vi "DimostratoreTest.vi"() -> ()   [LabVIEW 2019]
doc: "Dimostratore API\n\nFunzionamento:\n1. Seleziona postazione e data\n Conferma\n Ottieni un array con tutti i test della postazione selezionata in base alla data\n2. Seleziona quale test eseguire\n Conferma che tutti gli assets dei test sono disponibili\n Mostra tutti gli step di un test\n3. Seleziona Step da eseguire inserendo anche un valore di prova\n Il risultato dello step viene riprodotto nell'outcome\n\nFunzionamento alternativo\n1. Imposta uno Step Id e conferma\n2. Inserisci un valore di prova e ottieni l'outcome"
uses:
  ByteGSAPIBase/ByteGSAPIBase.lvclass
  TypeDef/MachineStates.ctl
  ByteGSAPIBase/TypeDef/Test.ctl
  ByteGSAPIBase/TypeDef/Asset.ctl
  ByteGSAPIBase/TypeDef/Step.ctl
  <vilib>/Utility/miscctls.llb/LVStringsAndValuesArrayTypeDef_I32.ctl
panel:
  in  "Exit":bool=TRUE
  out "Step Name":string
  in  "Home":bool
  in  "Indietro":bool
  out "Infos":string
  in  "Duration":dbl
  in  "Ottieni Passaggio Step":bool
  in  "Step Id":i32
  in  "Valore Prova":dbl
  in  "Inizia Step":bool
  in  "Seleziona Step":i32(ring) items=["Prova di durata"=23]
  in  "Inizia Test":bool
  in  "Seleziona Test":i32(ring)
  out "error out":errorcluster
  in  "error in (no error)":errorcluster
  in  "Ottieni Test Per Postazione":bool
  in  "ByteGSAPIBase in":refnum<class "ByteGSAPIBase.lvclass">
  in  "Data Partenza":timestamp format="%<%x>T"
  in  "Postazione":enum16{"POST 1", "POST 2"}(ring)
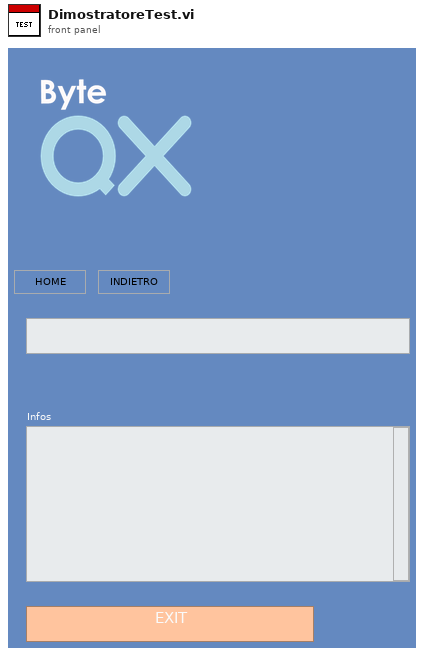
[diagram p1: front panel]
types:
  T1 = typedef "ByteGSWebAPI.lvlib/ByteGSAPIBase.lvclass/Step.ctl" = cluster{"id":i32, "descrizione":string, "prova":string, "assets":T2[], "criterio_accettazione":string, "valore_criterio_accettazione_max":dbl, "valore_criterio_accettazione_min":dbl, "udm_criterio_accettazione":string, "duration_prova":string, "udm_duration_prova":string, "valore_prova":dbl, "ordine":i32, "user":i32, "link_automation":string, "instruction_automation":string, "data_completamento_checklist":timestamp, "outcome":bool}
  T2 = typedef "ByteGSWebAPI.lvlib/ByteGSAPIBase.lvclass/Asset.ctl" = cluster{"descrizione":string, "slug":string, "id":i32}
  T3 = typedef "ByteGSWebAPI.lvlib/ByteGSAPIBase.lvclass/Test.ctl" = cluster{"titolo":string, "descrizione":string, "statoprova":string, "assets":T2[], "id":i32, "data_apertura_prova":timestamp}
  T4 = typedef "MachineStates.ctl" = enum16{"Initialize", "Idle", "GetLimsTestsForBench", "AssetsCheck", "GetLimsTestSteps", "UpdateLimsTestStep", "GetLimsTestStep", "Indietro", "UpdateLimsTestStepAutomation"}
  T5 = cluster{"Postazione":refnum<vi>, "Data Partenza":refnum<vi>, "Ottieni Test Per Postazione":refnum<vi>, "Step Id":refnum<vi>, "Ottieni Passaggio Step":refnum<vi>, "Seleziona Test":refnum<vi>, "Inizia Test":refnum<vi>, "Seleziona Step":refnum<vi>, "Valore Prova":refnum<vi>, "Inizia Step":refnum<vi>, "Infos":refnum<vi>, "Duration":refnum<vi>, "Step Name":refnum<vi>, "Exit":refnum<vi>}
  T6 = cluster{"ByteGSAPIBase in":refnum<class "ByteGSAPIBase.lvclass">, "Array dei Test":T3[], "Steps Array":T1[]}
  T7 = typedef "LVStringsAndValuesArrayTypeDef_I32.ctl" = cluster{"String":string, "Value":i32}[]
  T8 = cluster{"Postazione":enum16{"POST 1", "POST 2"}, "Data Partenza":timestamp, "Seleziona Test":i32, "Seleziona Step":i32, "Valore Prova":dbl, "Step Id":i32, "Duration":dbl}
  T9 = typedef "ByteGSWebAPI.lvlib/ByteGSAPIBase.lvclass/UpdateLimsTestStepData.ctl" = cluster{"outcome":bool, "data_completamento_checklist":timestamp, "udm_duration_prova":string, "valore_prova":dbl, "link_automation":string, "instruction_automation":string, "duration_prova":string}
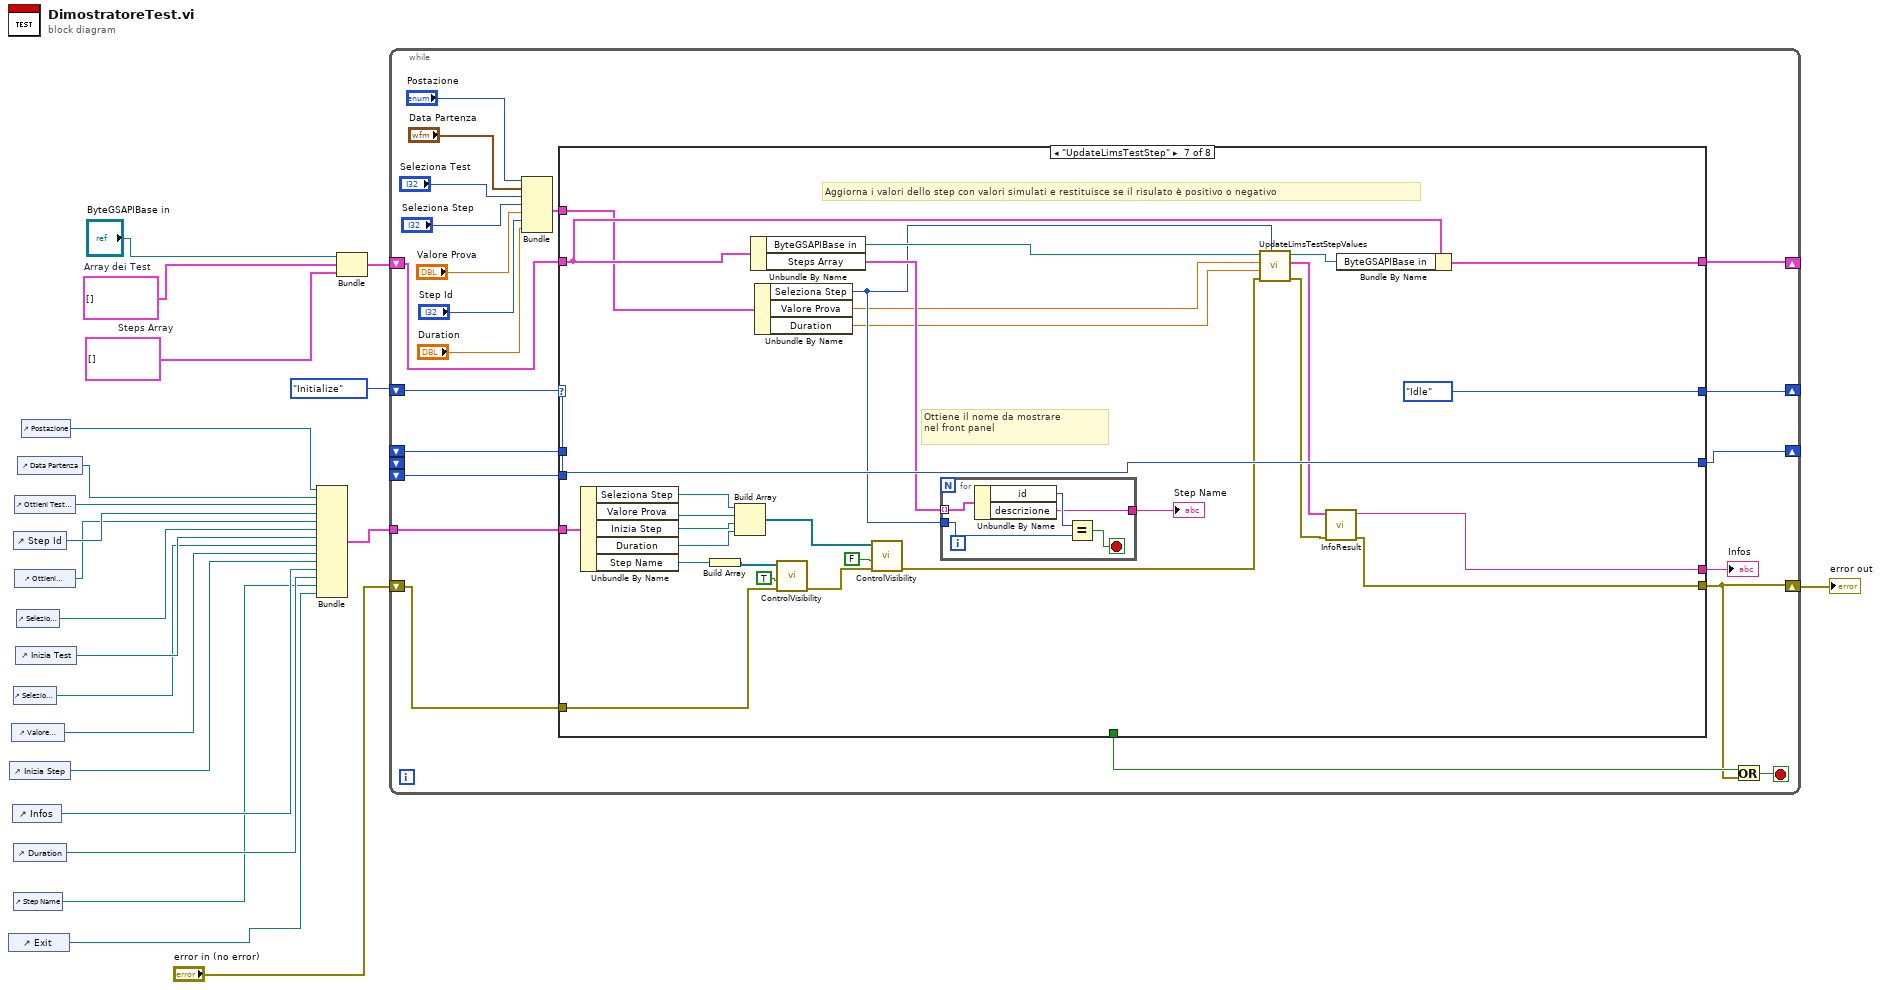
[diagram p0: block diagram]
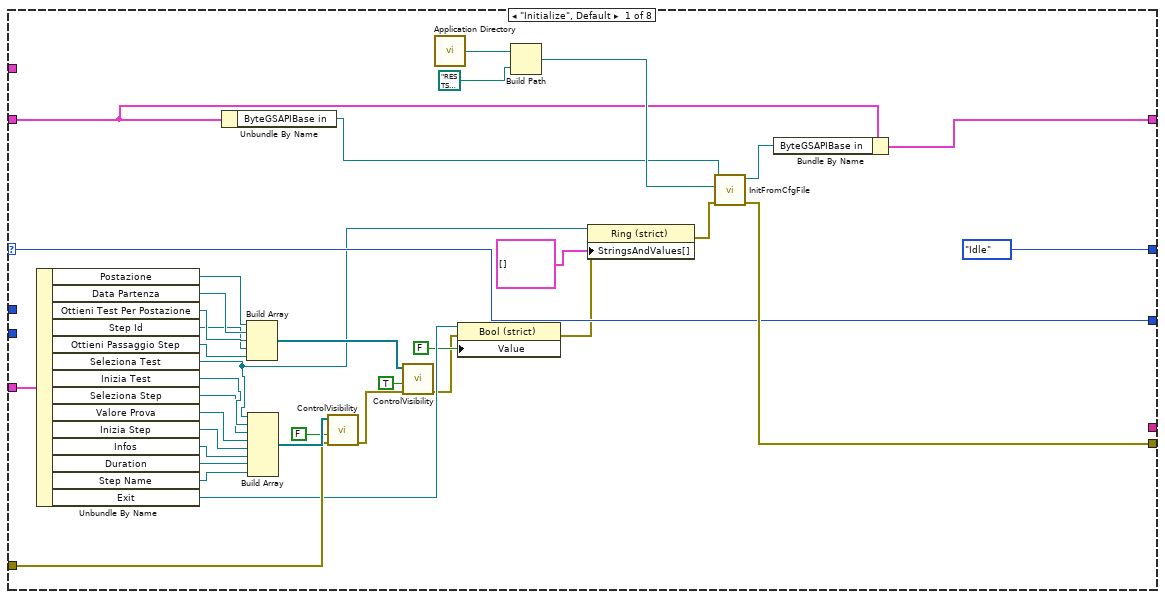
[diagram p2: hidden frame]
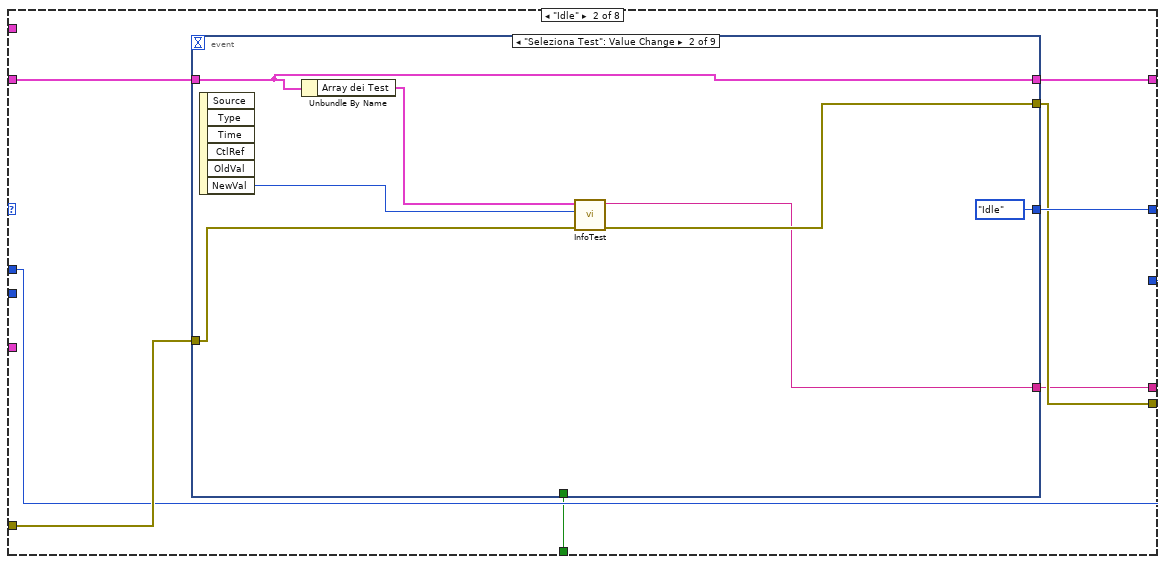
[diagram p3: hidden frame]
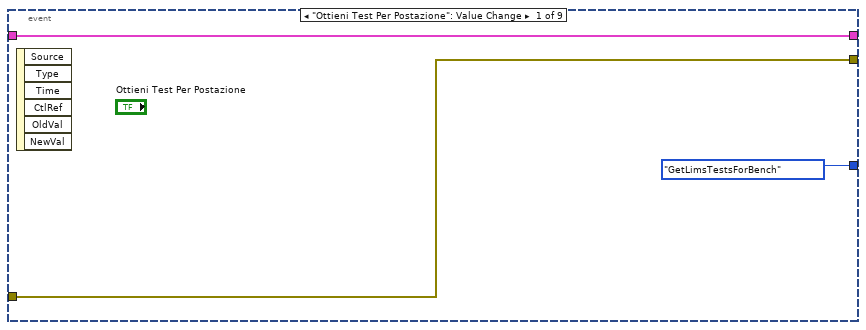
[diagram p4: hidden frame]
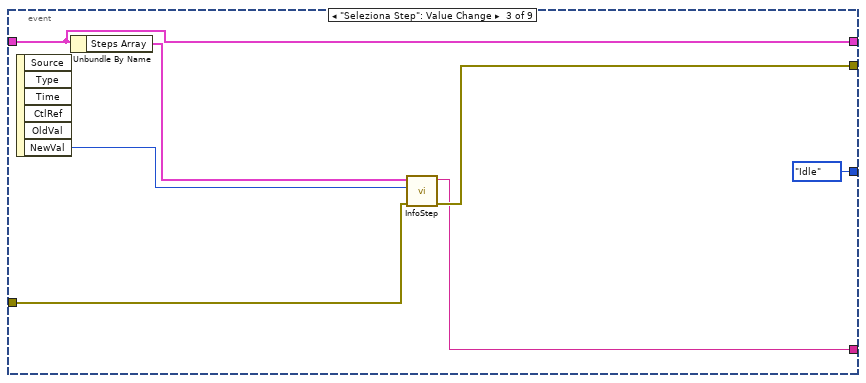
[diagram p5: hidden frame]
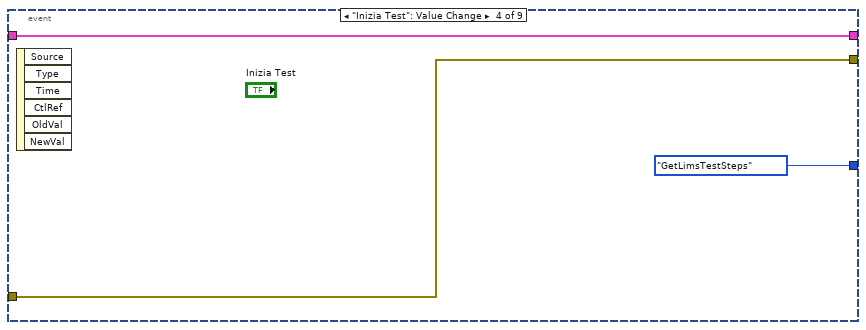
[diagram p6: hidden frame]
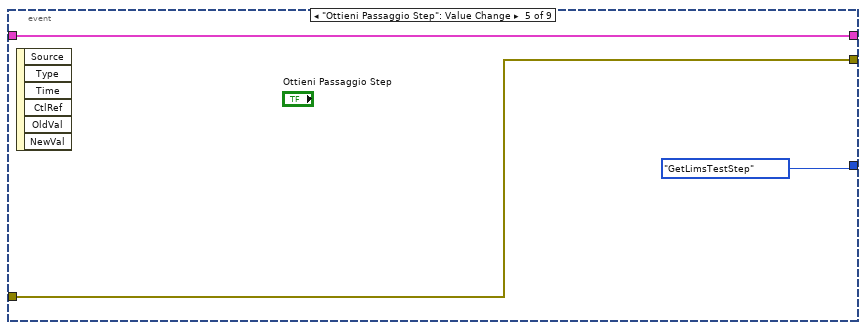
[diagram p7: hidden frame]
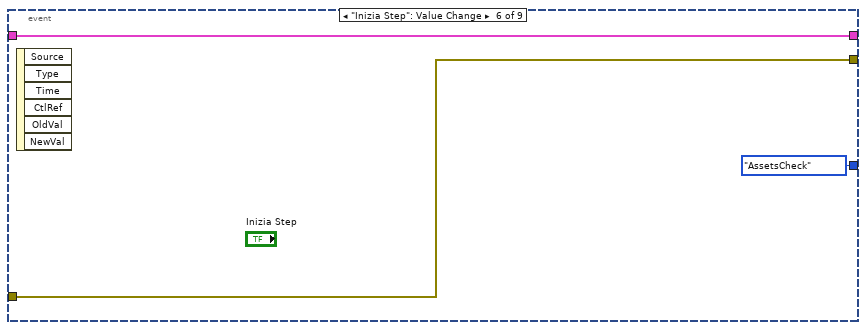
[diagram p8: hidden frame]
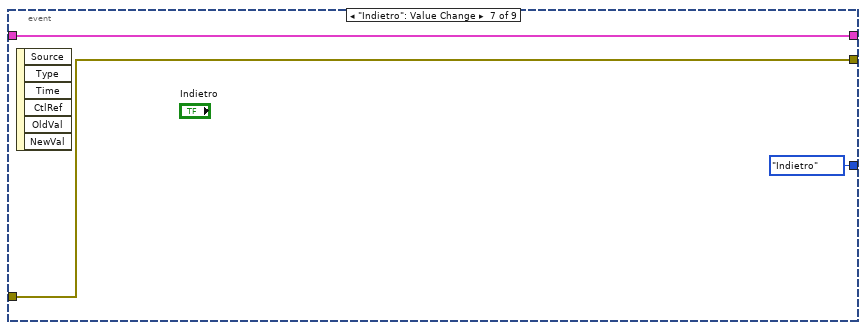
[diagram p9: hidden frame]
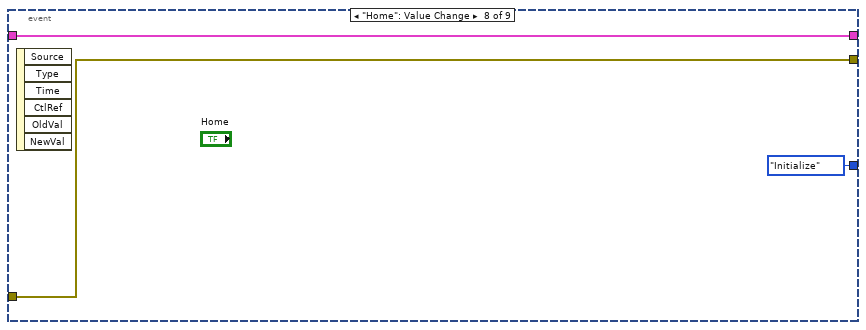
[diagram p10: hidden frame]
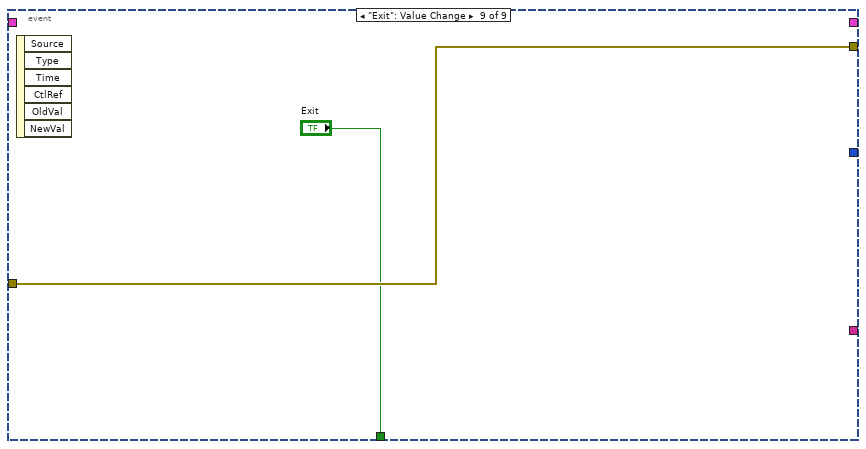
[diagram p11: hidden frame]
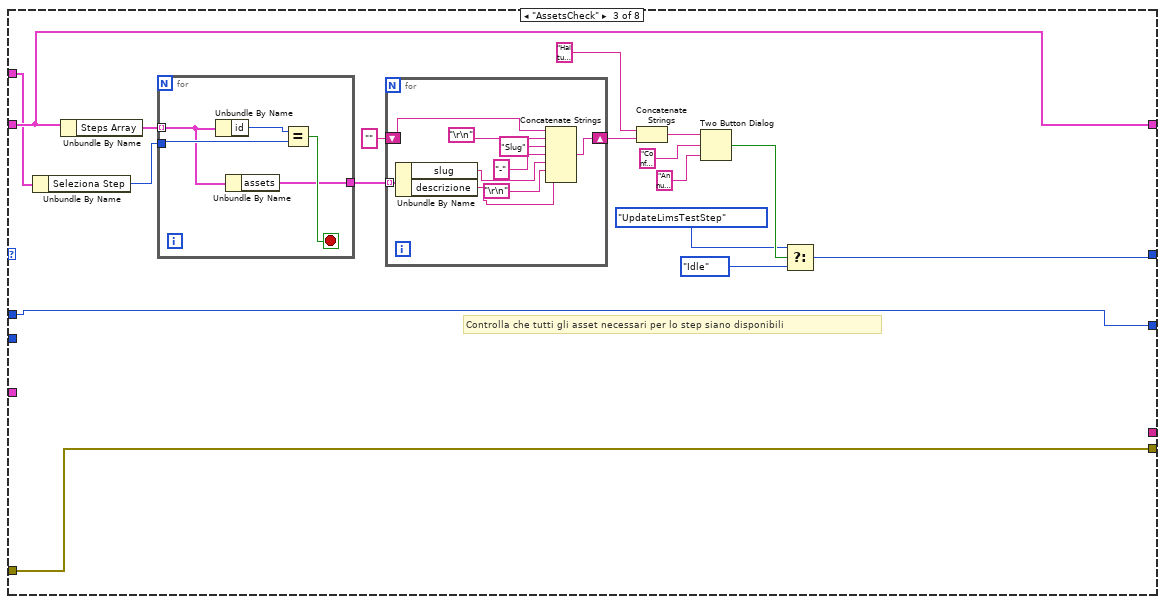
[diagram p12: hidden frame]
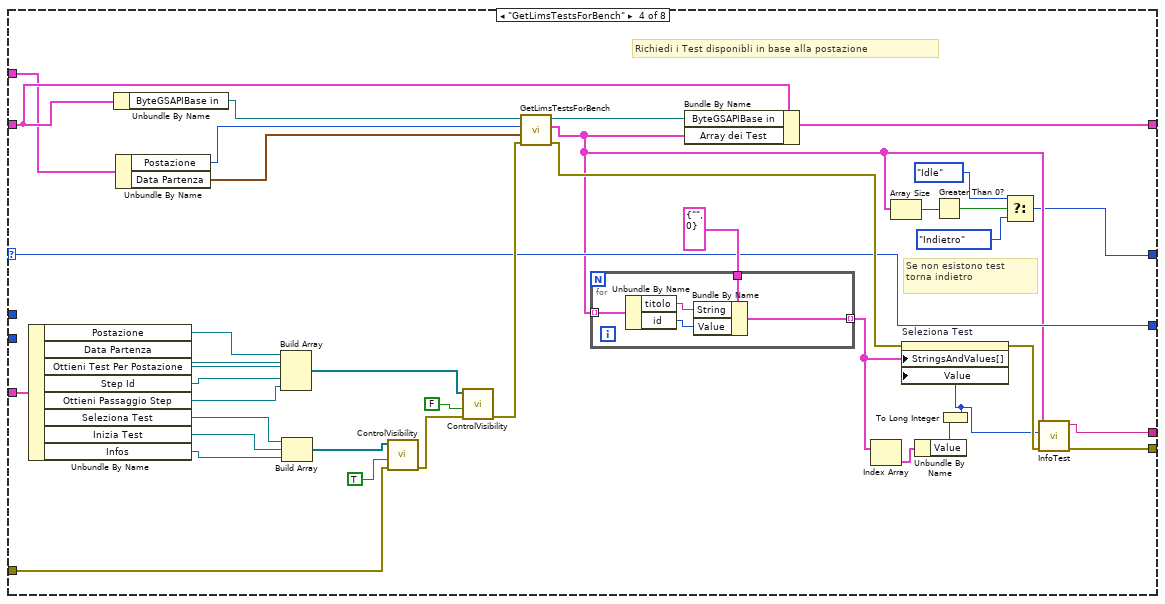
[diagram p13: hidden frame]
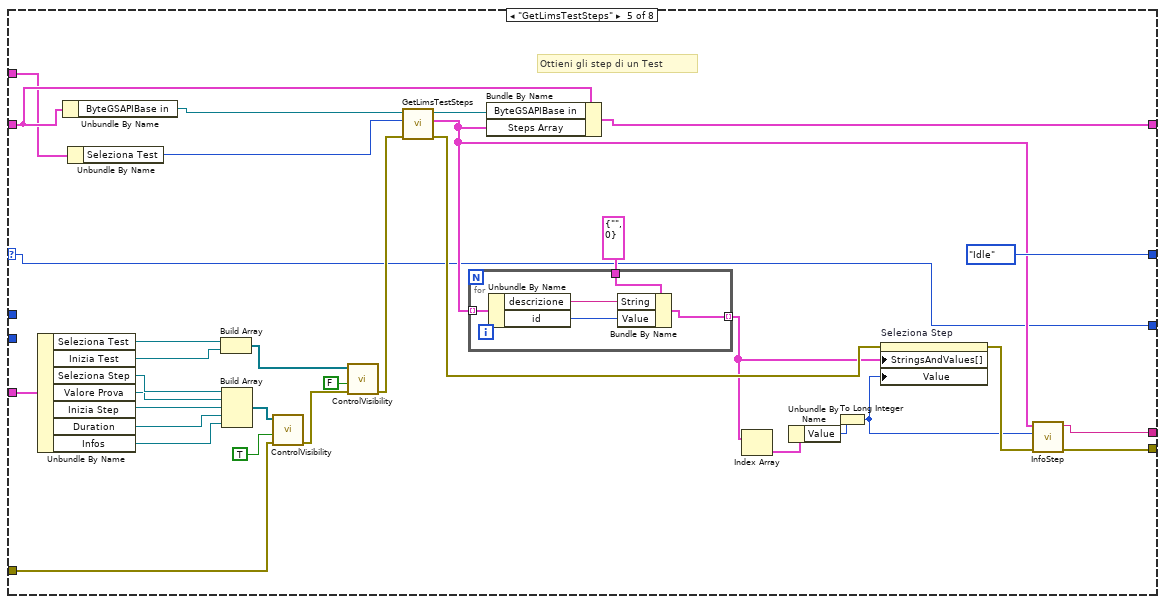
[diagram p14: hidden frame]
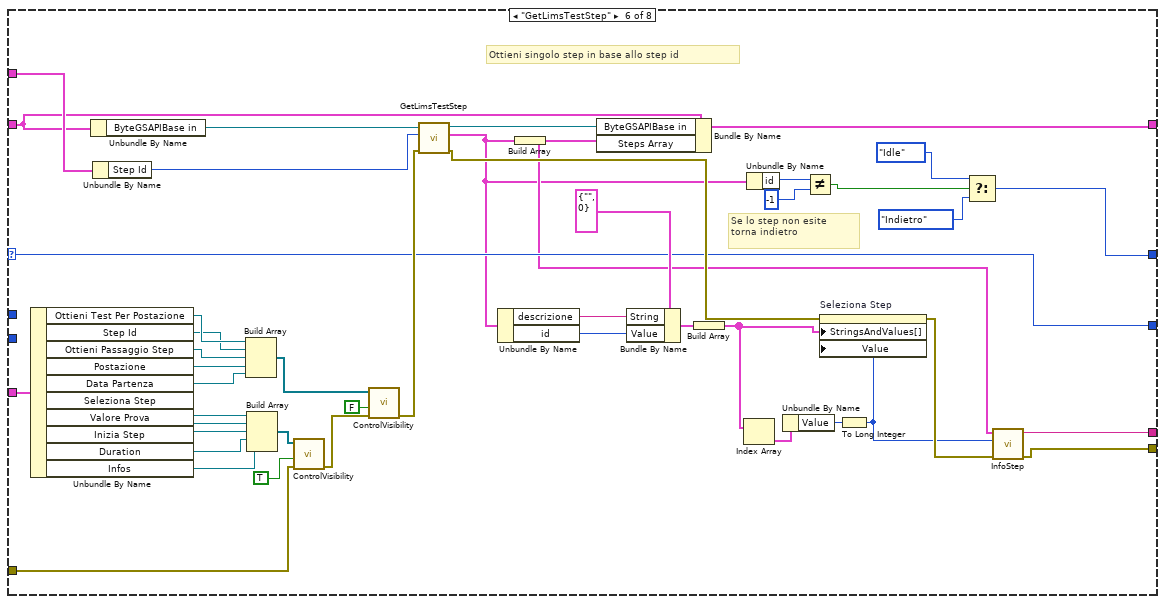
[diagram p15: hidden frame]
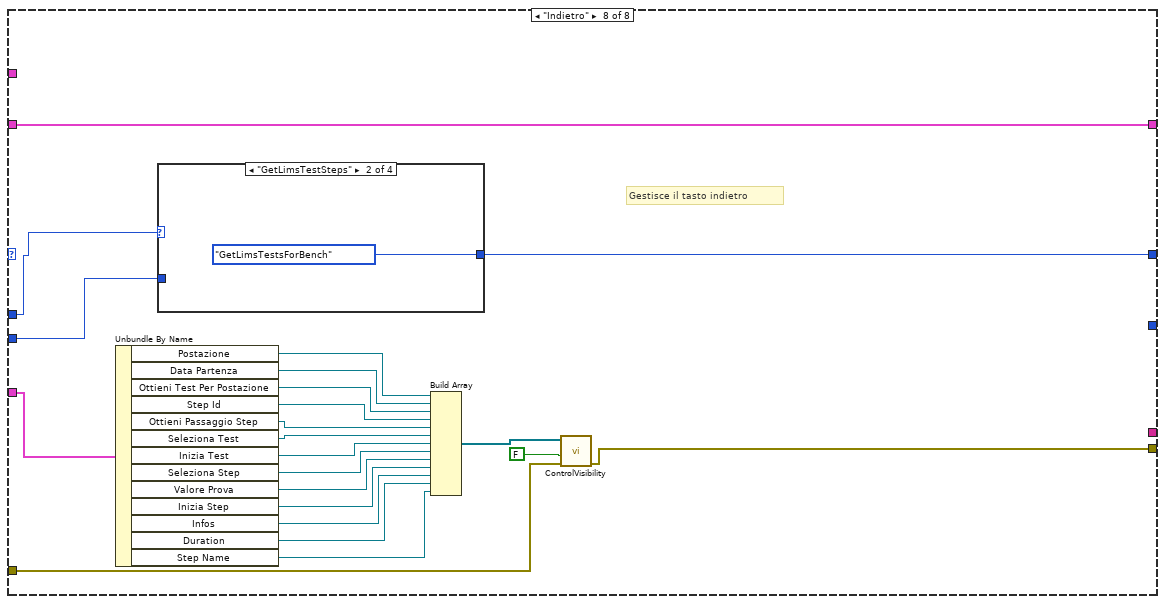
[diagram p16: hidden frame]
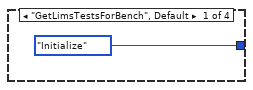
[diagram p17: hidden frame]
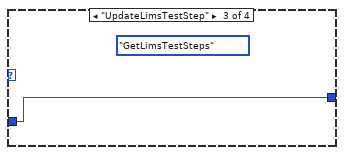
[diagram p18: hidden frame]
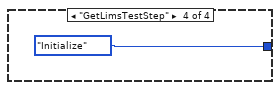
[diagram p19: hidden frame]
diagram:
  w19 = T1[] []  # Steps Array
  w21 = T3[] []  # Array dei Test
  n1 = control-ref of="Exit"() -> (w1:refnum<vi>)
  n2 = control-ref of="Inizia Step"() -> (w7:refnum<vi>)
  n3 = control-ref of="Valore Prova"() -> (w8:refnum<vi>)
  n4 = control-ref of="Infos"() -> (w3:refnum<vi>)
  n5 = control-ref of="Step Id"() -> (w13:refnum<vi>)
  n6 = control-ref of="Seleziona Step"() -> (w9:refnum<vi>)
  n7 = control-ref of="Duration"() -> (w5:refnum<vi>)
  n8 = control-ref of="Step Name"() -> (w2:refnum<vi>)
  n9 = control-ref of="Ottieni Test Per Postazione"() -> (w14:refnum<vi>)
  n10 = control-ref of="Ottieni Passaggio Step"() -> (w12:refnum<vi>)
  n11 = control-ref of="Inizia Test"() -> (w10:refnum<vi>)
  n12 = control-ref of="Seleziona Test"() -> (w11:refnum<vi>)
  n13 = control-ref of="Data Partenza"() -> (w15:refnum<vi>)
  n14 = control-ref of="Postazione"() -> (w16:refnum<vi>)
  n15 = Bundle("Postazione"=w16, "Data Partenza"=w15, "Ottieni Test Per Postazione"=w14, "Step Id"=w13, "Ottieni Passaggio Step"=w12, "Seleziona Test"=w11, "Inizia Test"=w10, "Seleziona Step"=w9, "Valore Prova"=w8, "Inizia Step"=w7, "Infos"=w3, "Duration"=w5, "Step Name"=w2, "Exit"=w1) -> (w6:T5)  [unwired: 1 in]
  n16 = Bundle("ByteGSAPIBase in"="ByteGSAPIBase in", "Array dei Test"=w21, "Steps Array"=w19) -> (w18:T6)  [unwired: 1 in]
  n17 = while {
    shift-right: [w42] -> _
    shift-left: MachineStates."Initialize" -> [w43]
    shift-right: [w41] -> _
    shift-left: w18 -> [w26]
    shift-right: [w24] -> w17
    shift-left: "error in (no error)" -> [w40]
    tunnel: w6 -> [w32]
    shift-right: [w30] -> _
    shift-left: _ -> [w29]
    shift-left: _ -> [_]
    shift-left: _ -> [w28]
    stop <- w23 stop-if-true
    n18 = Bundle("Postazione"="Postazione", "Data Partenza"="Data Partenza", "Seleziona Test"="Seleziona Test", "Seleziona Step"="Seleziona Step", "Valore Prova"="Valore Prova", "Step Id"="Step Id", "Duration"="Duration") -> (w34:T8)  [unwired: 1 in]
    n19 = case shown="\"UpdateLimsTestStep\"" w43 {
      selector: w43 -> [w52 _ _ w162 w200 w244 w302 _]
      tunnel: [MachineStates."Idle" w87 w129 w156 MachineStates."Idle" w240 MachineStates."Idle" w316] -> w42
      tunnel: w26 -> [w74 w86 w136 w191 w228 w275 w307 w335]
      tunnel: [w72 w85 w136 w190 w227 w276 w305 w335] -> w41
      tunnel: w40 -> [w55 w84 w138 w163 w207 w251 w285 w319]
      tunnel: [w71 w83 w138 w180 w205 w248 w300 w318] -> w24
      tunnel: w34 -> [_ _ w125 w186 w221 w279 w303 _]
      tunnel: w32 -> [w70 _ _ w166 w216 w255 w297 w325]
      tunnel: [_ w82 _ w179 w206 w247 w299 _] -> w27
      tunnel: [w52 w81 w122 w162 w200 w244 w302 _] -> w30
      tunnel: w29 -> [_ w81 w122 _ _ _ _ w317]
      tunnel: w28 -> [_ _ _ _ _ _ _ w315]
      tunnel: [_ w80 _ _ _ _ _ _] -> w25
      frame "Initialize", Default {
        n20 = Unbundle By Name(w70) -> ("Postazione"=w64:refnum<vi>, "Data Partenza"=w63:refnum<vi>, "Ottieni Test Per Postazione"=w62:refnum<vi>, "Step Id"=w61:refnum<vi>, "Ottieni Passaggio Step"=w60:refnum<vi>, "Seleziona Test"=w50:refnum<vi>, "Inizia Test"=w69:refnum<vi>, "Seleziona Step"=w68:refnum<vi>, "Valore Prova"=w67:refnum<vi>, "Inizia Step"=w66:refnum<vi>, "Infos"=w65:refnum<vi>, "Duration"=w53:refnum<vi>, "Step Name"=w51:refnum<vi>, "Exit"=w48:refnum<vi>)
        n21 = Unbundle By Name(w74) -> ("ByteGSAPIBase in"=w75:refnum<class "ByteGSAPIBase.lvclass">)
        n22 = Build Array(w64, w63, w62, w61, w60) -> (w58:refnum<vi>[])
        n23 = Build Array(w50, w69, w68, w67, w66, w65, w53, w51) -> (w59:refnum<vi>[])
        n24 = call "ControlVisibility.vi"("error in (no error)"=w55, "Visible"=FALSE, "Controls"=w59) -> ("error out"=w54:errorcluster)  [unwired: 8 in]
        n25 = call "ControlVisibility.vi"("error in (no error)"=w54, "Visible"=TRUE, "Controls"=w58) -> ("error out"=w45:errorcluster)  [unwired: 8 in]
        n26 = call <vilib>:"Application Directory.vi"() -> ("Application Directory"=w77:path)
        n27 = property class="Bool (strict)"(reference=w48, error in=w45, "Value"=FALSE) -> (error out=w46:errorcluster)  [unwired: 1 out]
        n28 = Build Path(base path=w77, name or relative path=path "RESTServerCfg_LIMS.ini") -> (appended path=w78:path)
        n29 = property class="Ring (strict)"(reference=w50, error in=w46, "StringsAndValues[]"=T7 [] ("Strings And Values []")) -> (error out=w49:errorcluster)  [unwired: 1 out]
        n30 = call-dynamic "InitFromCfgFile.vi"("error in (no error)"=w49, "configuration file path"=w78, "ByteGSAPIBase in"=w75) -> ("error out"=w71:errorcluster, "ByteGSAPIBase out"=w73:refnum<class "ByteGSAPIBase.lvclass">)  [unwired: 7 in]
        n31 = Bundle By Name(cluster=w74, "ByteGSAPIBase in"=w73) -> (w72:T6)
      }
      frame "Idle" {
        n32 = event shown="[1] \"Seleziona Test\": Value Change" {
          selector: _ -> [_ _ _ _ _ _ _ _ _]
          dyn-events: _ -> [_ _ _ _ _ _ _ _ _]
          timeout: _ -> [_ _ _ _ _ _ _ _ _]
          tunnel: [MachineStates."GetLimsTestsForBench" MachineStates."Idle" MachineStates."Idle" MachineStates."GetLimsTestSteps" MachineStates."GetLimsTestStep" MachineStates."AssetsCheck" MachineStates."Indietro" MachineStates."Initialize" _] -> w87
          tunnel: w86 -> [w88 w97 w103 w106 w110 w113 w115 w118 _]
          tunnel: [w88 w97 w103 w106 w110 w113 w115 w118 _] -> w85
          tunnel: w84 -> [w89 w96 w99 w105 w109 w112 w116 w119 w121]
          tunnel: [w89 w95 w101 w105 w109 w112 w116 w119 w121] -> w83
          tunnel: [_ w93 w100 _ _ _ _ _ _] -> w82
          tunnel: [_ _ _ _ _ _ _ _ "Exit"] -> w80
          event "Ottieni Test Per Postazione": Value Change {
            n33 = event-data() -> ()  [unwired: 1 in, 6 out]
          }
          event "Seleziona Test": Value Change {
            n34 = event-data() -> ("NewVal"=w91:i32)  [unwired: 1 in, 5 out]
            n35 = Unbundle By Name(w97) -> ("Array dei Test"=w92:T3[])
            n36 = call "InfoTest.vi"("error in"=w96, "Seleziona Test"=w91, "TestForBenchArray"=w92) -> ("error out"=w95:errorcluster, "Info Test"=w93:string)  [unwired: 7 in]
          }
          event "Seleziona Step": Value Change {
            n37 = event-data() -> ("NewVal"=w98:i32)  [unwired: 1 in, 5 out]
            n38 = Unbundle By Name(w103) -> ("Steps Array"=w104:T1[])
            n39 = call "InfoStep.vi"("error in"=w99, "Seleziona Step"=w98, "Test Steps List"=w104) -> ("error out"=w101:errorcluster, "Info Test"=w100:string)  [unwired: 7 in]
          }
          event "Inizia Test": Value Change {
            n40 = event-data() -> ()  [unwired: 1 in, 6 out]
          }
          event "Ottieni Passaggio Step": Value Change {
            n41 = event-data() -> ()  [unwired: 1 in, 6 out]
          }
          event "Inizia Step": Value Change {
            n42 = event-data() -> ()  [unwired: 1 in, 6 out]
          }
          event "Indietro": Value Change {
            n43 = event-data() -> ()  [unwired: 1 in, 6 out]
          }
          event "Home": Value Change {
            n44 = event-data() -> ()  [unwired: 1 in, 6 out]
          }
          event "Exit": Value Change {
            n45 = event-data() -> ()  [unwired: 1 in, 6 out]
          }
        }
      }
      frame "AssetsCheck" {
        # "Controlla che tutti gli asset necessari per lo step siano disponibili"
        n46 = Unbundle By Name(w125) -> ("Seleziona Step"=w124:i32)
        n47 = Unbundle By Name(w136) -> ("Steps Array"=w137:T1[])
        n48 = for {
          tunnel: w137 -> [w149] mode=indexing
          tunnel: w124 -> [w151]
          tunnel: [w148] -> w135
          stop <- w150 stop-if-true
          n49 = Unbundle By Name(w149) -> ("id"=w152:i32)
          n50 = Unbundle By Name(w149) -> ("assets"=w148:T2[])
          n51 = Equal?(x=w152, y=w151) -> (x = y?=w150:bool)
        }
        n52 = for {
          tunnel: w135 -> [w146] mode=indexing
          shift-right: [w147] -> w134
          shift-left: "" -> [w145]
          n53 = Unbundle By Name(w146) -> ("slug"=w140:string, "descrizione"=w139:string)
          n54 = Concatenate Strings(w145, "\r\n", "Slug" ("string"), "-", w140, "\r\n", w139) -> (w147:string)
        }
        n55 = Concatenate Strings("Hai tutti gli assets per completare il Test?", w134) -> (w132:string)
        n56 = Two Button Dialog(message=w132, 1:"Annulla" ("F button name (\"Cancel\")"), 2:"Conferma" ("T button name (\"OK\")")) -> (T button?=w128:bool)
        n57 = Select(t=MachineStates."UpdateLimsTestStep", s=w128, f=MachineStates."Idle") -> (s? t:f=w129:T4)
      }
      frame "GetLimsTestsForBench" {
        # "Se non esistono test \ntorna indietro"
        # "Richiedi i Test disponibli in base alla postazione"
        n58 = Unbundle By Name(w166) -> ("Postazione"=w176:refnum<vi>, "Data Partenza"=w175:refnum<vi>, "Ottieni Test Per Postazione"=w174:refnum<vi>, "Step Id"=w173:refnum<vi>, "Ottieni Passaggio Step"=w172:refnum<vi>, "Seleziona Test"=w178:refnum<vi>, "Inizia Test"=w177:refnum<vi>, "Infos"=w165:refnum<vi>)
        n59 = Unbundle By Name(w191) -> ("ByteGSAPIBase in"=w185:refnum<class "ByteGSAPIBase.lvclass">)
        n60 = Unbundle By Name(w186) -> ("Postazione"=w154:enum16{"POST 1", "POST 2"}, "Data Partenza"=w153:timestamp)
        n61 = Build Array(w176, w175, w174, w173, w172) -> (w170:refnum<vi>[])
        n62 = Build Array(w178, w177, w165) -> (w171:refnum<vi>[])
        n63 = call "ControlVisibility.vi"("error in (no error)"=w163, "Visible"=TRUE, "Controls"=w171) -> ("error out"=w167:errorcluster)  [unwired: 8 in]
        n64 = call "ControlVisibility.vi"("error in (no error)"=w167, "Visible"=FALSE, "Controls"=w170) -> ("error out"=w164:errorcluster)  [unwired: 8 in]
        n65 = call-dynamic "GetLimsTestsForBench.vi"("error in (no error)"=w164, "Data Partenza"=w153, "Postazione"=w154, "ByteGSAPIBase in"=w185) -> ("error out"=w184:errorcluster, "Tests for bench"=w160:T3[], "ByteGSAPIBase out"=w183:refnum<class "ByteGSAPIBase.lvclass">)  [unwired: 5 in]
        n66 = for {
          tunnel: w160 -> [w196] mode=indexing
          tunnel: [w193] -> w188 mode=indexing
          tunnel: cluster{"String":string, "Value":u16} {"String"="", "Value"=0} ("Cluster") -> [w192]
          n67 = Unbundle By Name(w196) -> ("titolo"=w195:string, "id"=w194:i32)
          n68 = Bundle By Name(cluster=w192, "String"=w195, "Value"=w194) -> (w193:cluster{"String":string, "Value":u16})
        }
        n69 = Bundle By Name(cluster=w191, "ByteGSAPIBase in"=w183, "Array dei Test"=w160) -> (w190:T6)
        n70 = Index Array(array=w188) -> (element=w187:cluster{"String":string, "Value":u16})  [unwired: 1 in]
        n71 = Array Size(array=w160) -> (size(s)=w159:i32)
        n72 = Unbundle By Name(w187) -> ("Value"=w182:u16)
        n73 = Greater Than 0?(x=w159) -> (x > 0?=w158:bool)
        n74 = To Long Integer(number=w182) -> (32bit integer=w161:i32)
        n75 = property on="Seleziona Test" class="Ring (strict)"(error in=w184, "StringsAndValues[]"=w188, "Value"=w161) -> (error out=w181:errorcluster)  [unwired: 1 in, 1 out]
        n76 = Select(t=MachineStates."Idle", s=w158, f=MachineStates."Indietro") -> (s? t:f=w156:T4)
        n77 = call "InfoTest.vi"("error in"=w181, "Seleziona Test"=w161, "TestForBenchArray"=w160) -> ("error out"=w180:errorcluster, "Info Test"=w179:string)  [unwired: 7 in]
      }
      frame "GetLimsTestSteps" {
        # "Ottieni gli step di un Test"
        n78 = Unbundle By Name(w216) -> ("Seleziona Test"=w215:refnum<vi>, "Inizia Test"=w214:refnum<vi>, "Seleziona Step"=w213:refnum<vi>, "Valore Prova"=w212:refnum<vi>, "Inizia Step"=w211:refnum<vi>, "Duration"=w201:refnum<vi>, "Infos"=w199:refnum<vi>)
        n79 = Unbundle By Name(w228) -> ("ByteGSAPIBase in"=w229:refnum<class "ByteGSAPIBase.lvclass">)
        n80 = Unbundle By Name(w221) -> ("Seleziona Test"=w220:i32)
        n81 = Build Array(w215, w214) -> (w210:refnum<vi>[])
        n82 = Build Array(w213, w212, w211, w201, w199) -> (w209:refnum<vi>[])
        n83 = call "ControlVisibility.vi"("error in (no error)"=w207, "Visible"=TRUE, "Controls"=w209) -> ("error out"=w217:errorcluster)  [unwired: 8 in]
        n84 = call "ControlVisibility.vi"("error in (no error)"=w217, "Visible"=FALSE, "Controls"=w210) -> ("error out"=w208:errorcluster)  [unwired: 8 in]
        n85 = call-dynamic "GetLimsTestSteps.vi"("error in (no error)"=w208, "Test-id"=w220, "ByteGSAPIBase in"=w229) -> ("error out"=w224:errorcluster, "Test Steps List"=w202:T1[], "ByteGSAPIBase out"=w197:refnum<class "ByteGSAPIBase.lvclass">)  [unwired: 6 in]
        n86 = for {
          tunnel: w202 -> [w234] mode=indexing
          tunnel: [w233] -> w222 mode=indexing
          tunnel: cluster{"String":string, "Value":u16} {"String"="", "Value"=0} ("Cluster") -> [w232]
          n87 = Unbundle By Name(w234) -> ("descrizione"=w231:string, "id"=w230:i32)
          n88 = Bundle By Name(cluster=w232, "String"=w231, "Value"=w230) -> (w233:cluster{"String":string, "Value":u16})
        }
        n89 = Bundle By Name(cluster=w228, "ByteGSAPIBase in"=w197, "Steps Array"=w202) -> (w227:T6)
        n90 = Index Array(array=w222) -> (element=w223:cluster{"String":string, "Value":u16})  [unwired: 1 in]
        n91 = Unbundle By Name(w223) -> ("Value"=w204:u16)
        n92 = To Long Integer(number=w204) -> (32bit integer=w198:i32)
        n93 = property on="Seleziona Step" class="Ring (strict)"(error in=w224, "StringsAndValues[]"=w222, "Value"=w198) -> (error out=w203:errorcluster)  [unwired: 1 in, 1 out]
        n94 = call "InfoStep.vi"("error in"=w203, "Seleziona Step"=w198, "Test Steps List"=w202) -> ("error out"=w205:errorcluster, "Info Test"=w206:string)  [unwired: 7 in]
      }
      frame "GetLimsTestStep" {
        # "Se lo step non esite \ntorna indietro"
        # "Ottieni singolo step in base allo step id"
        n95 = Unbundle By Name(w255) -> ("Ottieni Test Per Postazione"=w254:refnum<vi>, "Step Id"=w253:refnum<vi>, "Ottieni Passaggio Step"=w252:refnum<vi>, "Postazione"=w263:refnum<vi>, "Data Partenza"=w262:refnum<vi>, "Seleziona Step"=w261:refnum<vi>, "Valore Prova"=w260:refnum<vi>, "Inizia Step"=w259:refnum<vi>, "Duration"=w256:refnum<vi>, "Infos"=w245:refnum<vi>)
        n96 = Unbundle By Name(w275) -> ("ByteGSAPIBase in"=w278:refnum<class "ByteGSAPIBase.lvclass">)
        n97 = Unbundle By Name(w279) -> ("Step Id"=w277:i32)
        n98 = Build Array(w254, w253, w252, w263, w262) -> (w258:refnum<vi>[])
        n99 = Build Array(w261, w260, w259, w256, w245) -> (w257:refnum<vi>[])
        n100 = call "ControlVisibility.vi"("error in (no error)"=w251, "Visible"=TRUE, "Controls"=w257) -> ("error out"=w264:errorcluster)  [unwired: 8 in]
        n101 = call "ControlVisibility.vi"("error in (no error)"=w264, "Visible"=FALSE, "Controls"=w258) -> ("error out"=w250:errorcluster)  [unwired: 8 in]
        n102 = call-dynamic "GetLimsTestStep.vi"("error in (no error)"=w250, "Step-id"=w277, "ByteGSAPIBase in"=w278) -> ("error out"=w267:errorcluster, "StepList"=w238:T1, "ByteGSAPIBase out"=w274:refnum<class "ByteGSAPIBase.lvclass">)  [unwired: 6 in]
        n103 = Unbundle By Name(w238) -> ("descrizione"=w271:string, "id"=w272:i32)
        n104 = Build Array(w238) -> (w239:T1[])
        n105 = Bundle By Name(cluster=w275, "ByteGSAPIBase in"=w274, "Steps Array"=w239) -> (w276:T6)
        n106 = Bundle By Name(cluster=cluster{"String":string, "Value":u16} {"String"="", "Value"=0} ("Cluster"), "String"=w271, "Value"=w272) -> (w269:cluster{"String":string, "Value":u16})
        n107 = Build Array(w269) -> (w268:cluster{"String":string, "Value":u16}[])
        n108 = Index Array(array=w268) -> (element=w273:cluster{"String":string, "Value":u16})  [unwired: 1 in]
        n109 = Unbundle By Name(w238) -> ("id"=w237:i32)
        n110 = Unbundle By Name(w273) -> ("Value"=w246:u16)
        n111 = Not Equal?(x=w237, y=-1) -> (x != y?=w235:bool)
        n112 = To Long Integer(number=w246) -> (32bit integer=w243:i32)
        n113 = property on="Seleziona Step" class="Ring (strict)"(error in=w267, "StringsAndValues[]"=w268, "Value"=w243) -> (error out=w249:errorcluster)  [unwired: 1 in, 1 out]
        n114 = Select(t=MachineStates."Idle", s=w235, f=MachineStates."Indietro") -> (s? t:f=w240:T4)
        n115 = call "InfoStep.vi"("error in"=w249, "Seleziona Step"=w243, "Test Steps List"=w239) -> ("error out"=w248:errorcluster, "Info Test"=w247:string)  [unwired: 7 in]
      }
      frame "UpdateLimsTestStep" {
        # "Ottiene il nome da mostrare\nnel front panel"
        # "Aggiorna i valori dello step con valori simulati e restituisce se il risulato è positivo o negativo"
        n116 = Unbundle By Name(w297) -> ("Seleziona Step"=w295:refnum<vi>, "Valore Prova"=w294:refnum<vi>, "Inizia Step"=w293:refnum<vi>, "Duration"=w292:refnum<vi>, "Step Name"=w286:refnum<vi>)
        n117 = Build Array(w286) -> (w287:refnum<vi>[])
        n118 = Build Array(w295, w294, w293, w292) -> (w291:refnum<vi>[])
        n119 = Unbundle By Name(w307) -> ("ByteGSAPIBase in"=w308:refnum<class "ByteGSAPIBase.lvclass">, "Steps Array"=w290:T1[])
        n120 = Unbundle By Name(w303) -> ("Seleziona Step"=w283:i32, "Valore Prova"=w282:dbl, "Duration"=w281:dbl)
        n121 = call "ControlVisibility.vi"("error in (no error)"=w285, "Visible"=TRUE, "Controls"=w287) -> ("error out"=w284:errorcluster)  [unwired: 8 in]
        n122 = call "ControlVisibility.vi"("error in (no error)"=w284, "Visible"=FALSE, "Controls"=w291) -> ("error out"=w296:errorcluster)  [unwired: 8 in]
        n123 = for {
          tunnel: w283 -> [w312]
          tunnel: w290 -> [w313] mode=indexing
          tunnel: [w310] -> w289
          stop <- w309 stop-if-true
          n124 = Unbundle By Name(w313) -> ("id"=w311:i32, "descrizione"=w310:string)
          n125 = Equal?(x=w311, y=w312) -> (x = y?=w309:bool)
        }
        "Step Name" <- w289
        n126 = call-dynamic "UpdateLimsTestStepValues.vi"("step_id"=w283, "error in (no error)"=w296, "duration_hours"=w281, "value"=w282, "ByteGSAPIBase in"=w308) -> ("error out"=w301:errorcluster, "Result Step"=w280:T9, "ByteGSAPIBase out"=w306:refnum<class "ByteGSAPIBase.lvclass">)  [unwired: 4 in]
        n127 = call "InfoResult.vi"("error in"=w301, "Result Step"=w280) -> ("error out"=w300:errorcluster, "Info Test"=w299:string)  [unwired: 8 in]
        n128 = Bundle By Name(cluster=w307, "ByteGSAPIBase in"=w306) -> (w305:T6)
      }
      frame "Indietro" {
        # "Gestisce il tasto indietro"
        n129 = Unbundle By Name(w325) -> ("Postazione"=w320:refnum<vi>, "Data Partenza"=w321:refnum<vi>, "Ottieni Test Per Postazione"=w322:refnum<vi>, "Step Id"=w323:refnum<vi>, "Ottieni Passaggio Step"=w324:refnum<vi>, "Seleziona Test"=w334:refnum<vi>, "Inizia Test"=w333:refnum<vi>, "Seleziona Step"=w332:refnum<vi>, "Valore Prova"=w331:refnum<vi>, "Inizia Step"=w330:refnum<vi>, "Infos"=w329:refnum<vi>, "Duration"=w326:refnum<vi>, "Step Name"=w314:refnum<vi>)
        n130 = case shown="\"GetLimsTestSteps\"" w317 {
          tunnel: [MachineStates."Initialize" MachineStates."GetLimsTestsForBench" w338 MachineStates."Initialize"] -> w316
          tunnel: w315 -> [_ _ w338 _]
          frame "GetLimsTestsForBench", Default {
          }
          frame "GetLimsTestSteps" {
          }
          frame "UpdateLimsTestStep" {
            (unwired) MachineStates."GetLimsTestSteps"
          }
          frame "GetLimsTestStep" {
          }
        }
        n131 = Build Array(w320, w321, w322, w323, w324, w334, w333, w332, w331, w330, w329, w326, w314) -> (w328:refnum<vi>[])
        n132 = call "ControlVisibility.vi"("error in (no error)"=w319, "Visible"=FALSE, "Controls"=w328) -> ("error out"=w318:errorcluster)  [unwired: 8 in]
      }
    }
    "Infos" <- w27
    n133 = Or(x=w25, y=w24) -> (x .or. y?=w23:bool)
  }
  "error out" <- w17
